vi "One_Command(SubVI).vi"(7 "string to write":string="ATZ", 8 "error in (no error)":errorcluster, 9 "delay before read (ms)":u32=265, 10 "wbc":dbl=4.0, 11 "VISA resource name":refnum<visa-resource-name>="COM11") -> (0 "error out":errorcluster, 3 "read string":string)   [LabVIEW 2017]
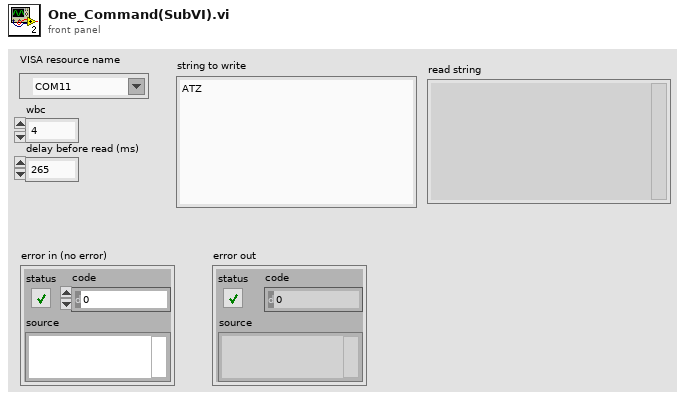
[diagram p1: front panel]
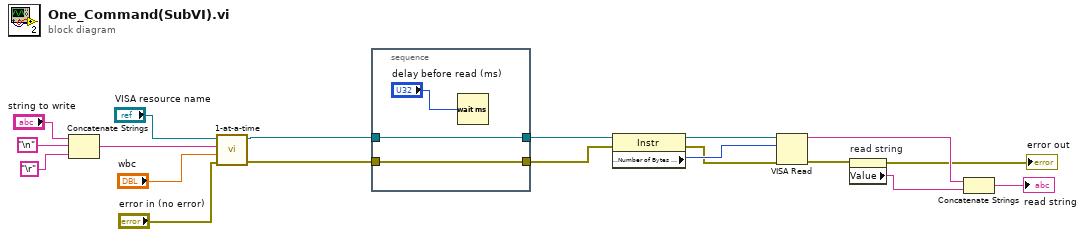
[diagram p0: block diagram]
diagram:
  n1 = Concatenate Strings("string to write", "\n", "\r") -> (w17:string)
  n2 = call "1-at-a-time.vi"("error in (no error)"="error in (no error)", "Wait Between Characters(ms)"="wbc", "write buffer"=w17, "VISA resource name"="VISA resource name") -> ("error out"=w13:errorcluster, "VISA resource name out"=w12:refnum<visa-resource-name>)  [unwired: 5 in, 1 out]
  n3 = stacked-sequence {
    tunnel: w13 -> [w22]
    tunnel: [w22] -> w18
    tunnel: w12 -> [w21]
    tunnel: [w21] -> w19
    frame #0 {
      n4 = Wait (ms)(milliseconds to wait="delay before read (ms)") -> ()  [unwired: 1 out]
    }
  }
  n5 = property class="Instr"(reference=w19, error in=w18) -> (reference out=w3:refnum<visa-resource-name>, error out=w4:errorcluster, "Serial Settings:Number of Bytes at Serial Port"=w5:u32)
  n6 = VISA Read(VISA resource name=w3, byte count=w5, error in (no error)=w4) -> (read buffer=w6:string, error out=w8:errorcluster)  [unwired: 2 out]
  n7 = property on="read string" class="Str"(error in=w8) -> (error out=→"error out":errorcluster, "Value"=w9:string)  [unwired: 1 in, 1 out]
  n8 = Concatenate Strings(w6, w9) -> (→"read string":string)
